vi "Get Attribute I32.vi"(8 "error in":errorcluster, 10 "Attribute":string, 11 "IConfigurable in":refnum<class "IConfigurable.lvclass">) -> (0 "error out":errorcluster, 2 "Value":i32, 3 "IConfigurable out":refnum<class "IConfigurable.lvclass">)   [LabVIEW 2024, in "IConfigurable.lvclass"]
uses:
  IConfigurable.lvclass
  IConfigure/IConfigure.lvclass
  IConfiguration/IConfiguration.lvclass
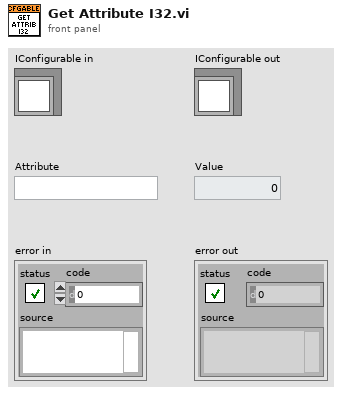
[diagram p1: front panel]
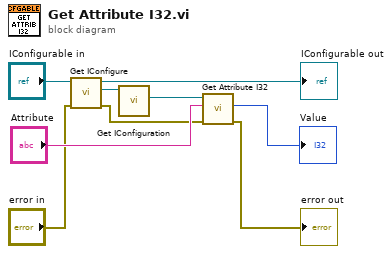
[diagram p0: block diagram]
diagram:
  n1 = call-dynamic "Get IConfigure.vi"("error in"="error in", "IConfigurable in"="IConfigurable in") -> ("error out"=w2:errorcluster, "IConfigure"=w5:refnum<class "IConfigure.lvclass">, "IConfigurable out"=→"IConfigurable out":refnum<class "IConfigurable.lvclass">)  [unwired: 7 in]
  n2 = call-dynamic "Get IConfiguration.vi"("IConfigure in"=w5) -> ("IConfiguration"=w4:refnum<class "IConfiguration.lvclass">)  [unwired: 9 in, 1 out]
  n3 = call-dynamic "Get Attribute I32.vi"("error in"=w2, "Attribute"="Attribute", "IConfiguration in"=w4) -> ("error out"=→"error out":errorcluster, "Value"=→"Value":i32)  [unwired: 6 in, 1 out]
